vi "SVFA Power Spectrum (1 Ch).vi"(0 "scaled signal [EU]":waveform(dbl), 2 "window":T8=1 items=["None"=0, "Hanning"=1, "Hamming"=2, "Blackman-Harris"=3, "Exact Blackman"=4, "Blackman"=5, "Flat Top"=6, "4 Term B-Harris "=7, "7 Term B-Harris"=8, "Low Sidelobe"=9, "Force"=64, "Exponential"=65, "Blackman Nuttall"=11, "Triangle"=30, "Bartlett-Hanning"=31, "Bohman"=32, "Parzen"=33, "Welch"=34, "Kaiser"=60, "Dolph-Chebyshev"=61, "Gaussian"=62], 4 "dB On (T)":bool=TRUE, 5 "error in (no error)":errorcluster, 7 "averaging parameters":T7={"averaging mode"=enum."No averaging", "weighting mode"=enum."Exponential", "number of averages"=10, "linear mode"=enum."One shot"}, 9 "restart averaging (F)":bool) -> (11 "averaging done":bool, 13 "averages completed":dbl, 14 "power spectrum [dB EU]":cluster{"f0":dbl, "df":dbl, "magnitude":dbl[]} {"magnitude" format="%.2p"; "df" format="%.2p"; "f0" format="%.2p"}, 15 "unit label":string, 18 "spectrum info":T1={"channel name"="", "description"="", "x-axis units"=0, "spectral info"={"spectrum type"=enum."Power [Magnitude^2]", "linear/dB"=enum."linear", "window"=0, "window size"=0, "FFT size"=0}, "engineering units"=0, "custom label"="", "dB reference [EU]"=0.0, "peak units"=enum."rms", "weighting filter"=0, "spectral density?"=FALSE, "unit label"="", "spectrum skewed?"=FALSE, "complimentary spectrum units"=enum."none"} {"x-axis units" items=["Time (s)"=0, "Frequency-CB (Hz)"=1, "Frequency-CPB (Hz)"=1248, "Frequency-Arbitrary (Hz)"=2357, "Quefrency (s)"=2, "Revolutions (rev)"=3, "Order"=4, "Speed (RPM)"=11, "Speed (rad/s)"=21, "Index"=65535]; "weighting filter" items=["Linear", "A-weighting", "B-weighting", "C-weighting", "ITU-R 468-4", "Dolby", "CCITT", "C-message", "Wb", "Wc", "Wd", "We", "Wf", "Wh", "Wj", "Wk", "Wm", "AES17 20 kHz lowpass", "AES17 40 kHz lowpass", "AES17 20 kHz highpass", "AES17 40 kHz highpass"]; "dB reference [EU]" format="%.2f"; "engineering units" items=["custom..."=0, "V"=1, "A"=21, "C"=30, "pC"=31, "s"=32, "-"=29, "Pa"=2, "N"=20, "g"=3, "m/s^2"=4, "m/s"=5, "m"=6, "mm/s"=12, "mm"=13, "micron/s"=14, "micron"=15, "in/s^2"=7, "in/s"=8, "in"=9, "mil/s"=10, "mil"=11, "rad/s^2"=16, "rad/s"=17, "rad"=18, "deg/s^2"=26, "deg/s"=27, "deg"=28, "RPM"=22, "cycle/s^2"=23, "Hz"=24, "cycle"=25, "strain"=19]; "spectral info"."window" items=["None "=0, "Hanning"=1, "Hamming"=2, "Blackman-Harris"=3, "Exact Blackman"=4, "Blackman"=5, "Flat Top"=6, "4 Term B-Harris "=7, "7 Term B-Harris"=8, "Low Sidelobe"=9, "Force - Exponential"=10, "Gaussian"=62]}, 19 "error out":errorcluster)   [LabVIEW 2017]
doc: "Computes the power spectrum of <B>scaled signal [EU]</B>. Use the power spectrum to quantify signal components as a function of frequency. Wire data to the <B>scaled signal [EU]</B> input to determine the polymorphic instance to use or manually select the instance."
uses:
  <vilib>/addons/_NISVFA/_Shared subVIs/Controls/svc_Window.ctl
  <vilib>/addons/_NISVFA/_Shared subVIs/Controls/svc_Spectrum Info.ctl
  <vilib>/addons/_NISVFA/_Shared subVIs/Controls/svc_X-Axis Units.ctl
  <vilib>/addons/_NISVFA/_Shared subVIs/Controls/svc_Spectrum Type.ctl
  <vilib>/addons/_NISVFA/_Shared subVIs/Controls/svc_Engineering Units Text Ring.ctl
  <vilib>/addons/_NISVFA/_Shared subVIs/Controls/svc_Weighting Filter Text Ring.ctl
  <vilib>/addons/_NISVFA/_Shared subVIs/Controls/svc_Complimentary Spectrum Units.ctl
  <vilib>/Analysis/2dsp.llb/Power Spectrum (DBL).vi
  <vilib>/Analysis/2dsp.llb/Real FFT.vi
  <vilib>/addons/_NISVFA/_Shared subVIs/Spectrum Averaging/svfa_No Average Array (complex).vi
  <vilib>/addons/_NISVFA/_Shared subVIs/Spectrum Averaging/svfa_Average Array (complex).vi
  <vilib>/addons/_NISVFA/_Shared subVIs/Common/svc_Get SV Channel Info.vi
  <vilib>/addons/_NISVFA/_Shared subVIs/Common/svc_Spectrum Units.vi
  <vilib>/addons/_NISVFA/_Shared subVIs/Windowing/svfa_Scaled Time Domain Window (Array).vi
  <vilib>/Analysis/4window.llb/Force Window.vi
  <vilib>/Analysis/4window.llb/Force Window (DBL).vi
  <vilib>/Analysis/4window.llb/Exponential Window.vi
  <vilib>/Analysis/4window.llb/Exponential Window (DBL).vi
  <vilib>/addons/_NISVFA/_Shared subVIs/Common/svc_Get Weighting Enum and Labels.vi
  <vilib>/addons/_NISVFA/_Shared subVIs/Common/svc_Unit Label Lexical Class.vi
  <vilib>/addons/_NISVFA/_Shared subVIs/Common/svc_Engineering Units to Unit Label.vi
  <vilib>/addons/_NISVFA/_Shared subVIs/Common/svc_Format Value (DBL).vi
  <vilib>/addons/_NISVFA/_Shared subVIs/Common/svc_Channel Info to Spectrum Info.vi
  <vilib>/addons/_NISVFA/_Shared subVIs/Common/svc_Unit Label to Engineering Units.vi
  <vilib>/Utility/error.llb/Error Cluster From Error Code.vi
  <vilib>/Analysis/0measdsp.llb/Scaled Time Domain Window.vi
  <vilib>/Analysis/0measdsp.llb/Scaled Time Domain Window (DBL).vi
  <vilib>/addons/_NISVFA/_Spectrum Processing/subVIs/svfa_Spectrum Info Window to windowTd Type Def.vi
  <vilib>/addons/_NISVFA/_Shared subVIs/Common/svc_Window Parameters.vi
  <vilib>/addons/_NISVFA/_Shared subVIs/Common/svc_Get Window Info.vi
  <vilib>/Analysis/NI_AALPro.lvlib
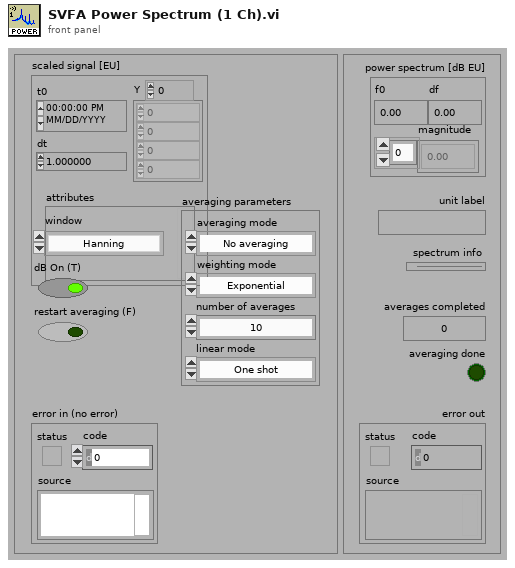
[diagram p1: front panel]
types:
  T1 = typedef "svc_Spectrum Info.ctl" = cluster{"channel name":string, "description":string, "x-axis units":T2, "spectral info":cluster{"spectrum type":T3, "linear/dB":enum16{"linear", "dB"}, "window":u16, "window size":i32, "FFT size":i32}, "engineering units":T4, "custom label":string, "dB reference [EU]":dbl, "peak units":enum16{"rms", "peak", "peak-peak"}, "weighting filter":T5, "spectral density?":bool, "unit label":string, "spectrum skewed?":bool, "complimentary spectrum units":T6}
  T2 = typedef "svc_X-Axis Units.ctl" = u16
  T3 = typedef "svc_Spectrum Type.ctl" = enum16{"FFT Spectrum [complex]", "Amplitude [Magnitude]", "Power [Magnitude^2]", "Cross Spectrum [complex]", "Frequency Response [Complex]"}
  T4 = typedef "svc_Engineering Units Text Ring.ctl" = u16
  T5 = typedef "svc_Weighting Filter Text Ring.ctl" = u16
  T6 = typedef "svc_Complimentary Spectrum Units.ctl" = enum16{"none", "radians", "degrees", "cycles", "imaginary"}
  T7 = cluster{"averaging mode":enum16{"No averaging", "Vector averaging", "RMS averaging", "Peak hold"}, "weighting mode":enum16{"Linear", "Exponential"}, "number of averages":u32, "linear mode":enum16{"One shot", "Auto restart"}}
  T8 = typedef "svc_Window.ctl" = u32
  T9 = enum16{"Restart processing", "Continue processing", "Skip processing"}
  T10 = cluster{"complex FFT":cdb[], "real FFT":dbl[], "f0":dbl, "df":dbl, "averages completed":dbl, "averaging parameters":cluster{"averaging mode":enum16{"No averaging", "Vector averaging", "RMS averaging", "Peak hold"}, "weighting mode":enum16{"Linear", "Exponential"}, "number of averages":u32, "linear mode":enum16{"One shot", "Auto restart"}}}
  T11 = enum16{"No averaging", "Vector averaging", "RMS averaging", "Peak hold"}
  T12 = cluster{"complex FFT":cdb[], "Mag/Real FFT":dbl[], "f0":dbl, "df":dbl, "averages completed":dbl, "averaging parameters":cluster{"averaging mode":enum16{"No averaging", "Vector averaging", "RMS averaging", "Peak hold"}, "weighting mode":enum16{"Linear", "Exponential"}, "number of averages":u32, "linear mode":enum16{"One shot", "Auto restart"}}}
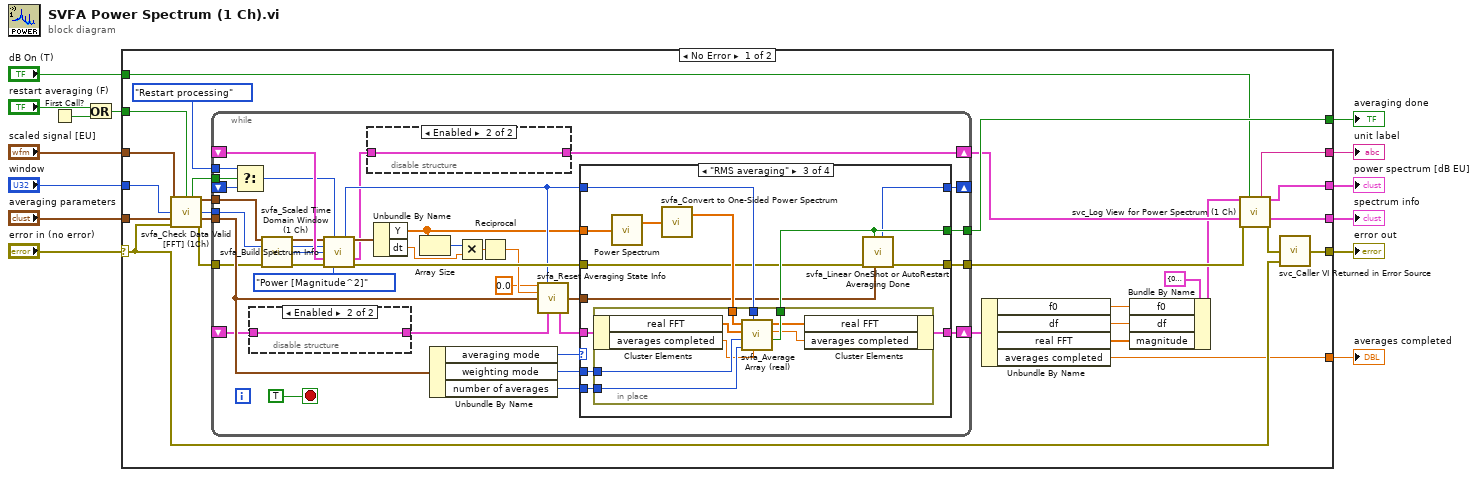
[diagram p0: block diagram]
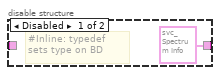
[diagram p2: hidden frame]
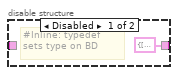
[diagram p3: hidden frame]
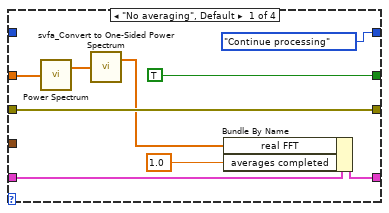
[diagram p4: hidden frame]
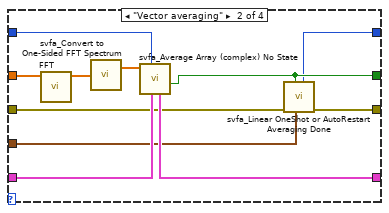
[diagram p5: hidden frame]
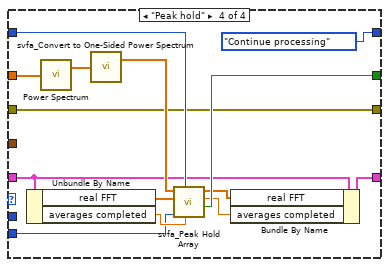
[diagram p6: hidden frame]
diagram:
  n1 = First Call?() -> (First Call?: T/F=w3:bool)
  n2 = Or(x="restart averaging (F)", y=w3) -> (x .or. y?=w1:bool)
  n3 = case shown="No Error" "error in (no error)" {
    selector: "error in (no error)" -> [w36 w139]
    tunnel: "scaled signal [EU]" -> [w39 _]
    tunnel: w1 -> [w40 _]
    tunnel: [w37 w139] -> w13
    tunnel: "averaging parameters" -> [w41 _]
    tunnel: "window" -> [w38 _]
    tunnel: [w22 _] -> w9
    tunnel: [w28 _] -> w8
    tunnel: "dB On (T)" -> [w26 _]
    tunnel: [w20 _] -> w6
    tunnel: [w27 _] -> w5
    tunnel: [w31 _] -> w4
    frame No Error {
      n4 = call <vilib>:"svfa_Check Data Valid [FFT] (1Ch).vi"("signal in [X]"=w39, "restart averaging (F)"=w40, "window"=w38, "averaging parameters"=w41, "error in (no error)"=w36) -> ("restart averaging"=w29:bool, "dup signal in [X]"=w32:waveform(dbl), "dup window"=w35:T8, "dup averaging parameters"=w33:T7, "error out"=w34:errorcluster)  [unwired: 6 in]
      n5 = while {
        tunnel: w35 -> [w73]
        shift-left: _ -> [w46]
        shift-right: [w66] -> w21
        tunnel: [w77] -> w31
        tunnel: [w65] -> w23
        tunnel: w33 -> [w78]
        tunnel: w34 -> [w75]
        shift-right: [w43] -> w25
        shift-left: _ -> [w72]
        shift-right: [w71] -> _
        shift-left: _ -> [w69]
        tunnel: w29 -> [w70]
        tunnel: T9."Restart processing" ("t") -> [w67]
        tunnel: w32 -> [w76]
        stop <- TRUE stop-if-true
        n6 = Select(t=w67, s=w70, f=w69) -> (s? t:f=w68:T9)
        n7 = disable-structure shown="Enabled" {
          disable-tunnel: [T10 {"complex FFT"=[], "real FFT"=[], "f0"=0.0, "df"=0.0, "averages completed"=0.0, "averaging parameters"={"averaging mode"=enum."No averaging", "weighting mode"=enum."Linear", "number of averages"=0, "linear mode"=enum."One shot"}} ("averaging state info out") w82] -> w45
          disable-tunnel: w46 -> [_ w82]
          frame Disabled {
            # "#Inline: typedef sets type on BD"
          }
          frame Enabled {
          }
        }
        n8 = call <vilib>:"svfa_Scaled Time Domain Window (1 Ch).vi"("Signal in [X]"=w76, "window"=w73, "error in"=w75) -> ("Windowed Waveform"=w58:waveform(dbl), "dup window"=w59:T8, "window length"=w53:i32, "error out"=w60:errorcluster)  [unwired: 7 in, 2 out]
        n9 = call <vilib>:"svfa_Build Spectrum Info.vi"("scaled signal [EU]"=w58, "processing control"=w68, "window"=w59, "window size"=w53, "spectrum info in"=w72, "error in (no error)"=w60, "spectrum type"=svc_Spectrum_Type."Power [Magnitude^2]") -> ("dup processing control"=w56:T9, "dup scaled signal [EU]"=w64:waveform(dbl), "spectrum info out"=w44:T1, "error out"=w62:errorcluster)  [unwired: 5 in]
        n10 = disable-structure shown="Enabled" {
          disable-tunnel: [T1 {"channel name"="", "description"="", "x-axis units"=0, "spectral info"={"spectrum type"=enum."Power [Magnitude^2]", "linear/dB"=enum."linear", "window"=0, "window size"=0, "FFT size"=0}, "engineering units"=1, "custom label"="", "dB reference [EU]"=0.0, "peak units"=enum."rms", "weighting filter"=0, "spectral density?"=FALSE, "unit label"="", "spectrum skewed?"=FALSE, "complimentary spectrum units"=enum."none"} ("spectrum info out") w80] -> w43
          disable-tunnel: w44 -> [_ w80]
          frame Disabled {
            # "#Inline: typedef sets type on BD"
          }
          frame Enabled {
          }
        }
        n11 = Unbundle By Name ("Get Waveform Components")(w64) -> ("Y"=w48:dbl[], "dt"=w54:dbl)
        n12 = Array Size(array=w48) -> (size(s)=w47:i32)
        n13 = Unbundle By Name(w78) -> ("averaging mode"=w63:T11, "weighting mode"=w51:enum16{"Linear", "Exponential"}, "number of averages"=w50:u32)
        n14 = Multiply(x=w47, y=w54) -> (x*y=w57:dbl)
        n15 = Reciprocal(x=w57) -> (1/x=w49:dbl)
        n16 = call <vilib>:"svfa_Reset Averaging State Info.vi"("f0"=0.0, "processing control"=w56, "df"=w49, "averaging parameters"=w78, "averaging state info in"=w45) -> ("dup averaging parameters"=w55:T7, "averaging state info out"=w52:T10)  [unwired: 9 in]
        n17 = case shown="\"RMS averaging\"" w63 {
          tunnel: [w88 w94 w106 w126] -> w65
          tunnel: [TRUE ("averaging done") w96 w109 w132] -> w77
          tunnel: w62 -> [w88 w92 w107 w126]
          tunnel: w55 -> [_ w95 w108 _]
          tunnel: w56 -> [_ w102 w110 w136]
          tunnel: w48 -> [w89 w100 w114 w137]
          tunnel: [w85 w97 w103 w128] -> w66
          tunnel: w52 -> [w86 w101 w104 w129]
          tunnel: w51 -> [_ _ w113 _]
          tunnel: w50 -> [_ _ w112 w133]
          tunnel: [T9."Continue processing" ("processing control") w93 w105 T9."Continue processing" ("processing control")] -> w71
          frame "No averaging", Default {
            n18 = call-poly <vilib>:"Power Spectrum.vi"("X"=w89) -> ("Power Spectrum"=w90:dbl[])  [unwired: 1 out]
            n19 = call <vilib>:"svfa_Convert to One-Sided Power Spectrum.vi"("two-sided power spectrum"=w90) -> ("one-sided power spectrum"=w84:dbl[])  [unwired: 1 out]
            n20 = Bundle By Name(cluster=w86, "real FFT"=w84, "averages completed"=1.0) -> (w85:T10)
          }
          frame "Vector averaging" {
            n21 = call-poly <vilib>:"FFT.vi"("X"=w100) -> ("FFT {X}"=w99:cdb[])  [unwired: 9 in, 1 out]
            n22 = call <vilib>:"svfa_Convert to One-Sided FFT Spectrum.vi"("two-sided FFT spectrum"=w99) -> ("one-sided FFT spectrum"=w98:cdb[])  [unwired: 1 out]
            n23 = call <vilib>:"svfa_Average Array (complex) No State.vi"("averaging state info in"=w101, "processing control"=w102, "array"=w98) -> ("averaging done"=w96:bool, "averaging state info out"=w97:T12)  [unwired: 5 in, 2 out]
            n24 = call <vilib>:"svfa_Linear OneShot or AutoRestart Averaging Done.vi"("averaging parameters"=w95, "averaging done"=w96, "error in (no error)"=w92) -> ("error out"=w94:errorcluster, "processing control"=w93:T9)  [unwired: 7 in]
          }
          frame "RMS averaging" {
            n25 = call-poly <vilib>:"Power Spectrum.vi"("X"=w114) -> ("Power Spectrum"=w115:dbl[])  [unwired: 1 out]
            n26 = call <vilib>:"svfa_Convert to One-Sided Power Spectrum.vi"("two-sided power spectrum"=w115) -> ("one-sided power spectrum"=w111:dbl[])  [unwired: 1 out]
            n27 = in-place {
              in-place-border: w113 -> [w124]
              in-place-border: w112 -> [w123]
              in-place-border: w111 -> [w122]
              in-place-border: w110 -> [w121]
              in-place-border: [w120] -> w109
              n28 = in-place-cluster #1(w104) -> ("real FFT"=w116:dbl[], "averages completed"=w119:dbl)
              n29 = call <vilib>:"svfa_Average Array (real).vi"("averages completed in"=w119, "processing control"=w121, "number of averages"=w123, "weighting mode"=w124, "previous average array"=w116, "array"=w122) -> ("averaging done"=w120:bool, "averages completed out"=w117:dbl, "average array"=w118:dbl[])  [unwired: 3 in]
              n30 = in-place-cluster #1("real FFT"=w118, "averages completed"=w117) -> (w103:T10)
            }
            n31 = call <vilib>:"svfa_Linear OneShot or AutoRestart Averaging Done.vi"("averaging parameters"=w108, "averaging done"=w109, "error in (no error)"=w107) -> ("error out"=w106:errorcluster, "processing control"=w105:T9)  [unwired: 7 in]
          }
          frame "Peak hold" {
            n32 = Unbundle By Name(w129) -> ("real FFT"=w135:dbl[], "averages completed"=w134:dbl)
            n33 = call-poly <vilib>:"Power Spectrum.vi"("X"=w137) -> ("Power Spectrum"=w138:dbl[])  [unwired: 1 out]
            n34 = call <vilib>:"svfa_Convert to One-Sided Power Spectrum.vi"("two-sided power spectrum"=w138) -> ("one-sided power spectrum"=w131:dbl[])  [unwired: 1 out]
            n35 = call <vilib>:"svfa_Peak Hold Array.vi"("averages completed in"=w134, "processing control"=w136, "number of averages"=w133, "previous peak array"=w135, "array"=w131) -> ("averaging done"=w132:bool, "averages completed out"=w130:dbl, "peak array"=w127:dbl[])  [unwired: 4 in]
            n36 = Bundle By Name(cluster=w129, "real FFT"=w127, "averages completed"=w130) -> (w128:T10)
          }
        }
      }
      n37 = Unbundle By Name(w21) -> ("f0"=w18:dbl, "df"=w17:dbl, "real FFT"=w16:dbl[], "averages completed"=w20:dbl)
      n38 = Bundle By Name(cluster=cluster{"f0":dbl, "df":dbl, "magnitude":dbl[]} {"f0"=0.0, "df"=0.0, "magnitude"=[]} ("power spectrum [dB EU]"), "f0"=w18, "df"=w17, "magnitude"=w16) -> (w15:cluster{"f0":dbl, "df":dbl, "magnitude":dbl[]})
      n39 = call <vilib>:"svc_Log View for Power Spectrum (1 Ch).vi"("power spectrum [dB EU]"=w15, "dB On (T)"=w26, "spectrum info"=w25, "error in (no error)"=w23) -> ("unit label"=w28:string, "power spectrum [dB EU]"=w22:cluster{"f0":dbl, "df":dbl, "magnitude":dbl[]}, "spectrum info out"=w27:T1, "error out"=w24:errorcluster)  [unwired: 8 in]
      n40 = call <vilib>:"svc_Caller VI Returned in Error Source.vi"("warning input to caller"=w36, "error in (no error)"=w24) -> ("error out"=w37:errorcluster)  [unwired: 3 in]
    }
    frame Error {
    }
  }
  "error out" <- w13
  "power spectrum [dB EU]" <- w9
  "unit label" <- w8
  "averaging done" <- w4
  "averages completed" <- w6
  "spectrum info" <- w5
